vi "3DM GX45 testing.vi"() -> ()   [LabVIEW 2011]
uses:
  Controls/Desciptor Set Byte.ctl
  <vilib>/robotics/Controls/Attitude Indicator/Attitude Indicator.xctl
  <vilib>/Instr/_visa.llb/VISA Configure Serial Port (Instr).vi
  SubVI/3DM-GX3-45 Commands/Start Stream.vi
  SubVI/3DM-GX3-45 Commands/Stop Stream.vi
panel:
  in  "VISA resource name":refnum<visa-resource-name>="COM5"
  out "Error Out":errorcluster
  in  "Error In":errorcluster
  out "Received array Size":i32
  out "YAW":dbl(knob) scale=-180.0..180.0
  out "Attitude Indicator":cluster{"Roll":dbl, "Pitch":dbl}(xcontrol)
  in  "Self Test":bool
  in  "Stop Data Stream":bool
  in  "Start Data Stream":bool
  out "Processing Loop Count":i32
  out "Received Array":u8[](array[numeric]) format="%02x"
  out "timed out?":bool
  out "Read Loop Count":i32
  in  "Field Data":u8[](array[numeric]) format="%02x"
  in  "Field Descriptor Byte":u8=117 format="%02x"
  in  "Data Set":T1=enum."NAV"
  out "result string":string
  out "Serial Settings:Number of Bytes at Serial Port":u32
  # "7565 0102 0205 E4CA”"
  # "7565 0102 027E 5D43”"
  # "desc"
  # "fld"
  # "desc"
  # "pld"
  # "----------ROLL-------------"
  # "----------Pitch-------------"
  # "----------Yaw-------------"
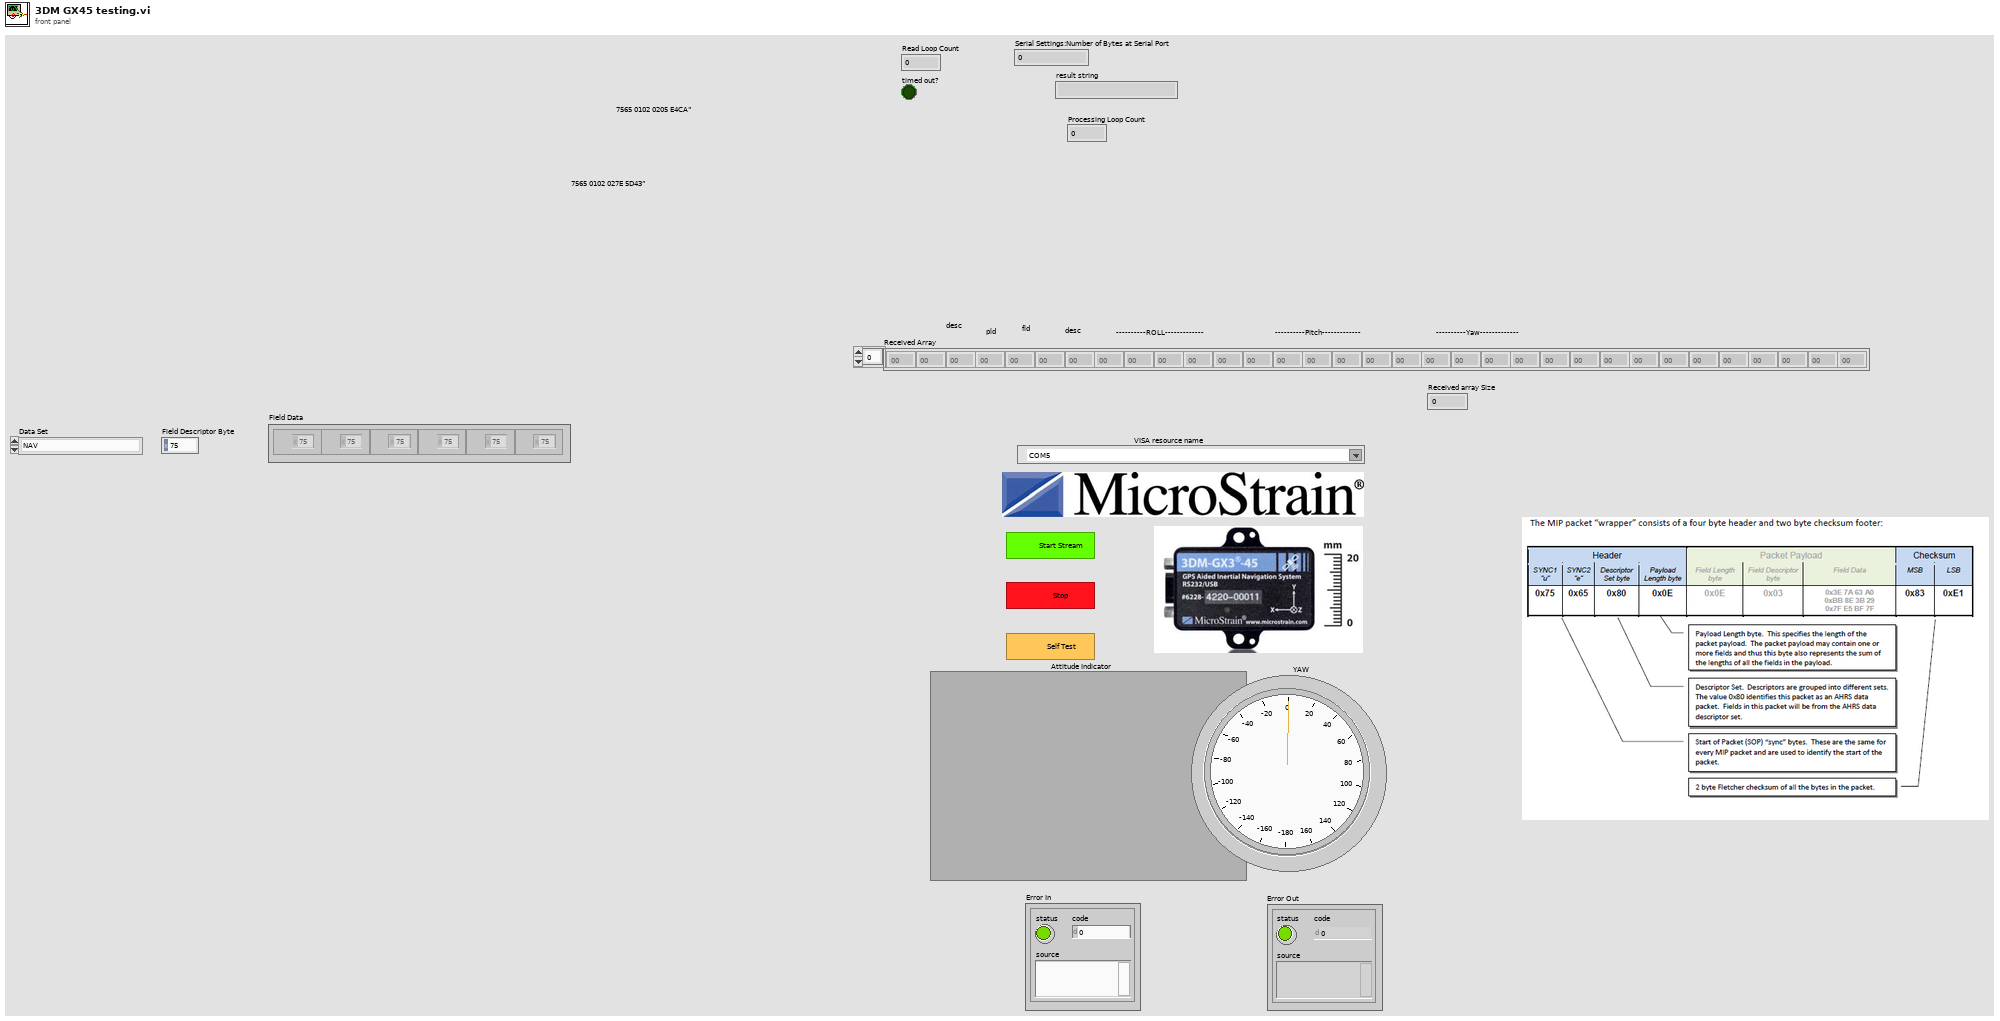
[diagram p1: front panel]
types:
  T1 = typedef "Desciptor Set Byte.ctl" = enum16{"Base Command Set", "3DM Command Set", "Navigation Filter Command Set", "System Command Set", "AHRS", "GPS", "NAV"}
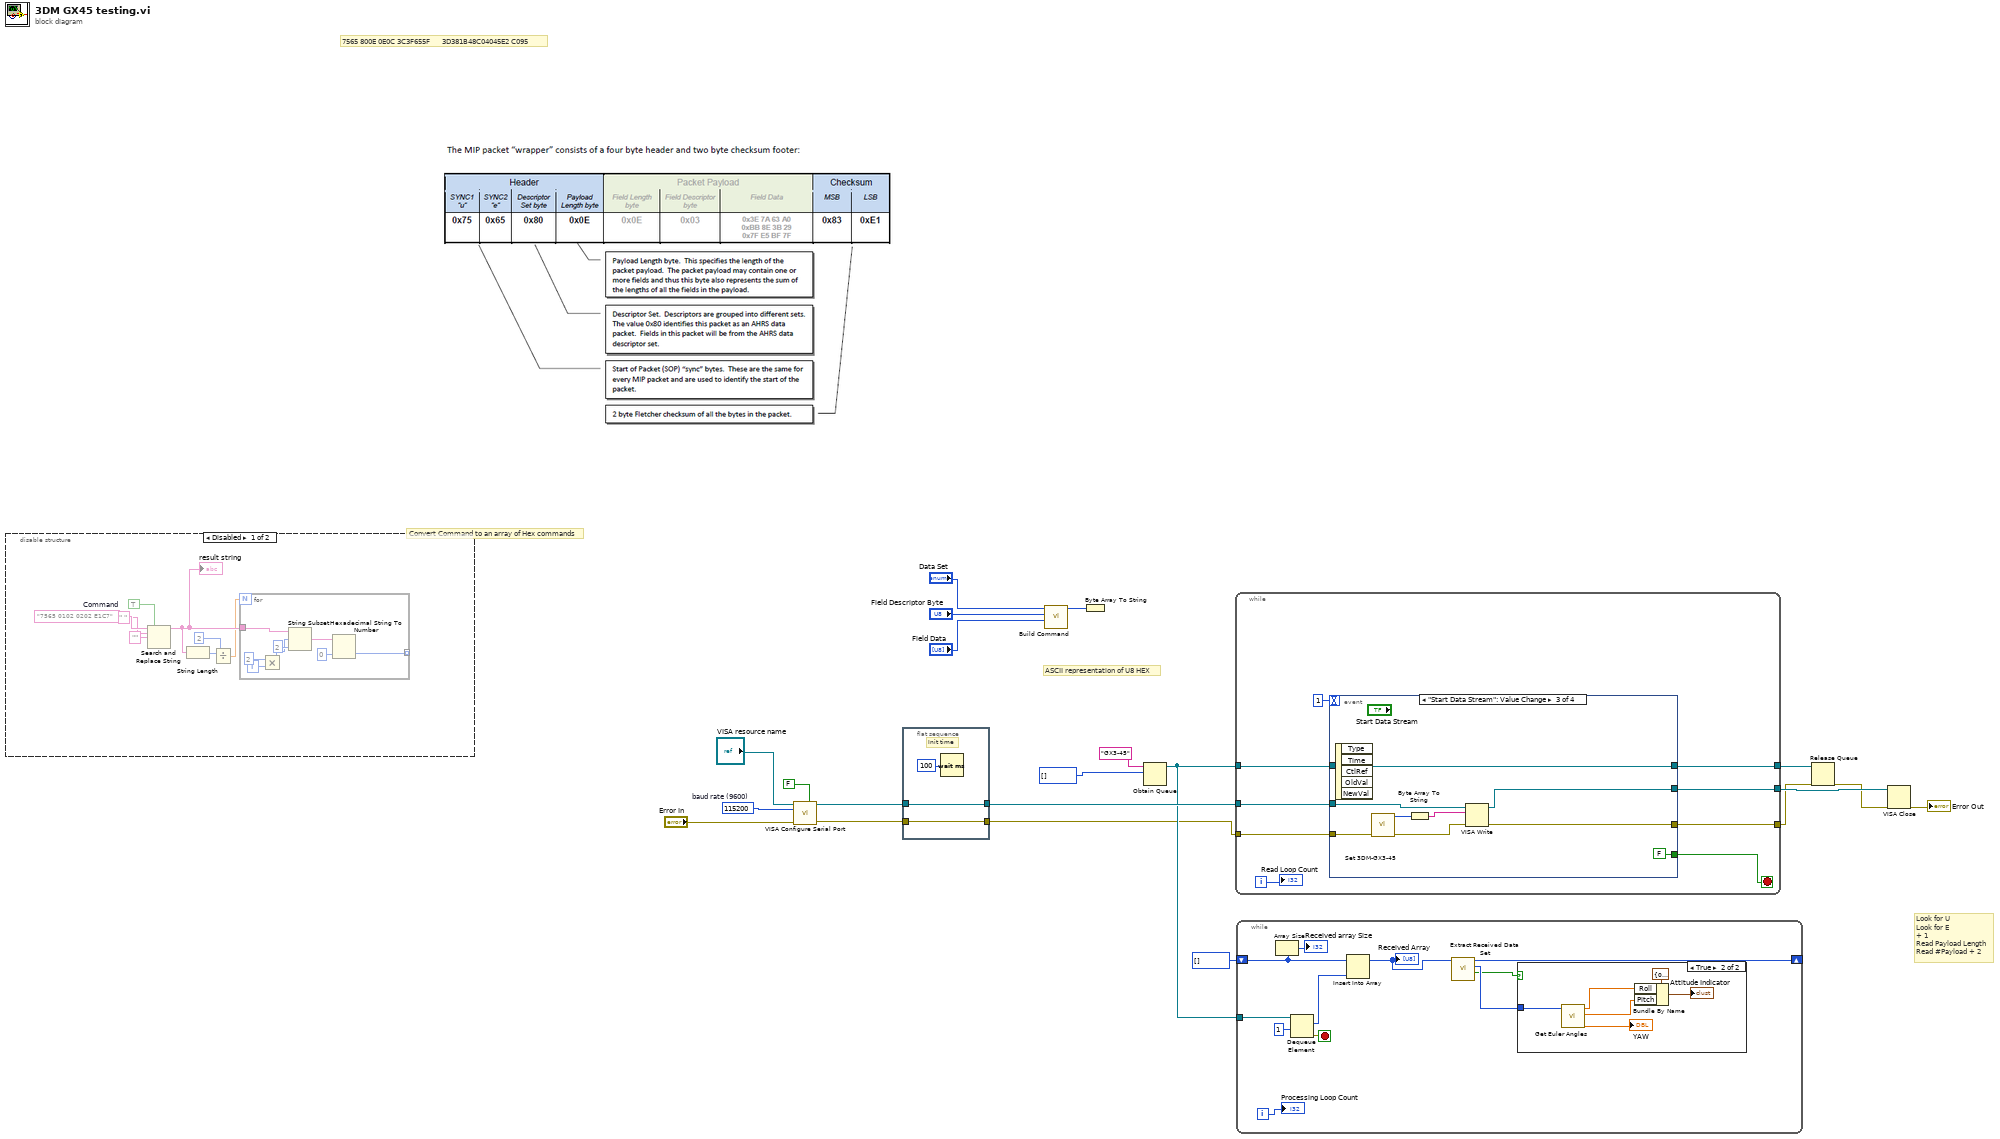
[diagram p0: block diagram]
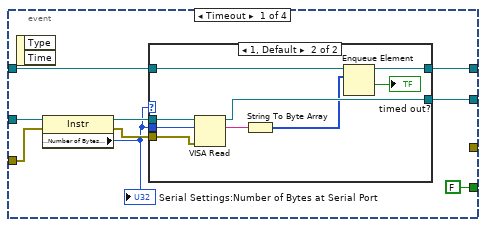
[diagram p4: hidden frame]
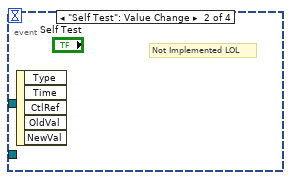
[diagram p6: hidden frame]
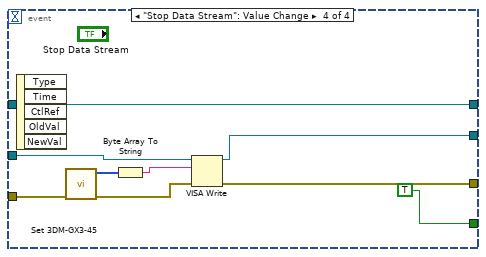
[diagram p7: hidden frame]
diagram:
  w17 = u32 115200  # baud rate (9600)
  # "7565 800E 0E0C 3C3F655F      3D381B48C04045E2 C095"
  # "Look for U\nLook for E\n+ 1\nRead Payload Length\nRead #Payload + 2"
  # "ASCII representation of U8 HEX"
  n1 = disable-structure shown="Disabled" {
    frame Disabled {
      w29 = "7565 0102 0202 E1C7"  # Command
      # "Convert Command to an array of Hex commands"
      n2 = Search and Replace String(replace all?=TRUE ("replace all? (F)"), input string=w29, search string=" ", replace string="" ("replace string (\"\")")) -> (result string=w25:string)  [unwired: 4 in, 3 out]
      "result string" <- w25
      n3 = String Length(string=w25) -> (length=w24:i32)
      n4 = Divide(x=w24, y=2) -> (x/y=w22:dbl)
      n5 = for {
        N: w22 -> [_]
        tunnel: w25 -> [w37]
        tunnel: [w30] -> _ mode=indexing
        i -> [w35]
        n6 = Multiply(x=2, y=w35) -> (x*y=w33:i32)
        n7 = String Subset(string=w37, offset (0)=w33, length (rest)=2 ("length (rest)")) -> (substring=w32:string)
        n8 = Hexadecimal String To Number(string=w32, default (0uL)=u8 0 ("default (0 U32)")) -> (number=w30:u8)  [unwired: 1 in, 1 out]
      }
    }
    frame Enabled {
    }
  }
  n9 = call-poly "VISA Configure Serial Port"("VISA resource name"="VISA resource name", "Enable Termination\nChar (T)"=FALSE ("Enable Termination\nChar (T)"), "baud rate (9600)"=w17, "error in (no error)"="Error In") -> ("VISA resource name out"=w7:refnum<visa-resource-name>, "error out"=w2:errorcluster)  [unwired: 10 in]
  n10 = flat-sequence {
    tunnel: w7 -> [w40]
    tunnel: [w40] -> w16
    tunnel: w2 -> [w38]
    tunnel: [w38] -> w1
    frame #0 {
      # "Init time"
      n11 = Wait (ms)(milliseconds to wait=u32 100) -> ()  [unwired: 1 out]
    }
  }
  n12 = call "Build Command.vi"("Field Data"="Field Data", "Field Descriptor Byte"="Field Descriptor Byte", "Data Set"="Data Set") -> ("Command"=w13:u8[])  [unwired: 7 in, 1 out]
  n13 = Byte Array To String(unsigned byte array=w13) -> ()  [unwired: 1 out]
  n14 = Obtain Queue(name (unnamed)="GX3-45", element data type=u8[] [] ("unsigned byte array")) -> (queue out=w10:refnum<queue>)  [unwired: 3 in, 2 out]
  n15 = while {
    tunnel: w16 -> [w49]
    tunnel: [w48] -> w14
    tunnel: w10 -> [w46]
    tunnel: [w45] -> w9
    tunnel: w1 -> [w43]
    tunnel: [w42] -> w6
    i -> [w47]
    stop <- w41 stop-if-true
    n16 = event shown="[2] \"Start Data Stream\": Value Change" {
      selector: _ -> [_ _ _ _]
      dyn-events: _ -> [_ _ _ _]
      timeout: 1 -> [_ _ _ _]
      tunnel: w49 -> [w58 _ w78 w87]
      tunnel: [w56 _ w75 w84] -> w48
      tunnel: w46 -> [w54 _ w70 w79]
      tunnel: [w52 _ w70 w79] -> w45
      tunnel: w43 -> [w51 _ w74 w83]
      tunnel: [_ _ w72 w81] -> w42
      tunnel: [FALSE ("Stop Data Stream 2") _ FALSE ("Stop Data Stream 2") TRUE ("Stop Data Stream 2")] -> w41
      event Timeout {
        n17 = event-data() -> ()  [unwired: 1 in, 2 out]
        n18 = property class="Instr"(reference=w58, error in=w51) -> (reference out=w57:refnum<visa-resource-name>, error out=w55:errorcluster, "Serial Settings:Number of Bytes at Serial Port"=w53:u32)
        "Serial Settings:Number of Bytes at Serial Port" <- w53
        n19 = case shown="1, Default" w53 {
          tunnel: w57 -> [w60 w69]
          tunnel: [w60 w68] -> w56
          tunnel: w53 -> [_ w67]
          tunnel: w55 -> [_ w66]
          tunnel: w54 -> [w59 w64]
          tunnel: [w59 w61] -> w52
          frame 0 {
          }
          frame 1, Default {
            n20 = VISA Read(VISA resource name=w69, byte count=w67, error in (no error)=w66) -> (VISA resource name out=w68:refnum<visa-resource-name>, read buffer=w65:string)  [unwired: 2 out]
            n21 = String To Byte Array(string=w65) -> (unsigned byte array=w63:u8[])
            n22 = Enqueue Element(queue=w64, element=w63) -> (queue out=w61:refnum<queue>, timed out?=→"timed out?":bool)  [unwired: 2 in, 1 out]
          }
        }
      }
      event "Self Test": Value Change {
        # "Not Implemented LOL"
        n23 = event-data() -> ()  [unwired: 1 in, 5 out]
      }
      event "Start Data Stream": Value Change {
        n24 = event-data() -> ()  [unwired: 1 in, 5 out]
        n25 = call-poly "Set 3DM-GX3-45.vi"("Error In"=w74) -> ("Error Out"=w73:errorcluster, "Command"=w77:u8[])  [unwired: 9 in]
        n26 = Byte Array To String(unsigned byte array=w77) -> (string=w76:string)
        n27 = VISA Write(VISA resource name=w78, write buffer=w76, error in (no error)=w73) -> (VISA resource name out=w75:refnum<visa-resource-name>, error out=w72:errorcluster)  [unwired: 1 out]
      }
      event "Stop Data Stream": Value Change {
        n28 = event-data() -> ()  [unwired: 1 in, 5 out]
        n29 = call-poly "Set 3DM-GX3-45.vi"("Error In"=w83) -> ("Error Out"=w82:errorcluster, "Command"=w86:u8[])  [unwired: 9 in]
        n30 = Byte Array To String(unsigned byte array=w86) -> (string=w85:string)
        n31 = VISA Write(VISA resource name=w87, write buffer=w85, error in (no error)=w82) -> (VISA resource name out=w84:refnum<visa-resource-name>, error out=w81:errorcluster)  [unwired: 1 out]
      }
    }
    "Read Loop Count" <- w47
  }
  n32 = while {
    tunnel: w10 -> [w98]
    shift-right: [w92] -> _
    shift-left: u8[] [] ("element") -> [w90]
    i -> [w95]
    stop <- w97 stop-if-true
    n33 = Array Size(array=w90) -> (size(s)=→"Received array Size":i32)
    n34 = Dequeue Element(queue=w98, timeout in ms (-1)=1) -> (element=w96:u8[], error out=w97:errorcluster)  [unwired: 1 in, 2 out]
    n35 = Insert Into Array(array=w90, new element=w96) -> (w94:u8[])  [unwired: 1 in]
    "Received Array" <- w94
    n36 = call "Extract Received Data Set.vi"("Received Array In"=w94) -> ("New Data Set Received"=w89:bool, "Extracted Data Set"=w93:u8[], "Received Array Out"=w92:u8[])  [unwired: 7 in, 1 out]
    n37 = case shown="True" w89 {
      tunnel: w93 -> [_ w104]
      frame False {
      }
      frame True {
        n38 = call "Get Euler Angles.vi"("Received Array"=w104) -> ("Yaw (deg)"=→"YAW":dbl, "Pitch (deg)"=w101:dbl, "Roll (deg)"=w99:dbl)  [unwired: 7 in]
        n39 = Bundle By Name(cluster=cluster{"Roll":dbl, "Pitch":dbl} {"Roll"=0.0, "Pitch"=0.0} ("Attitude Indicator 2"), "Roll"=w99, "Pitch"=w101) -> (→"Attitude Indicator":cluster{"Roll":dbl, "Pitch":dbl})
      }
    }
    "Processing Loop Count" <- w95
  }
  n40 = Release Queue(queue=w9, error in (no error)=w6) -> (error out=w5:errorcluster)  [unwired: 1 in, 2 out]
  n41 = VISA Close(VISA resource name=w14, error in (no error)=w5) -> (error out=→"Error Out":errorcluster)
